vi "acquire_2_b.vi"() -> ()   [LabVIEW 2023]
panel:
  in  "stop":bool
  out "Waveform Chart":i32(graph)
  out "error out":errorcluster
  in  "error in (no error)":errorcluster
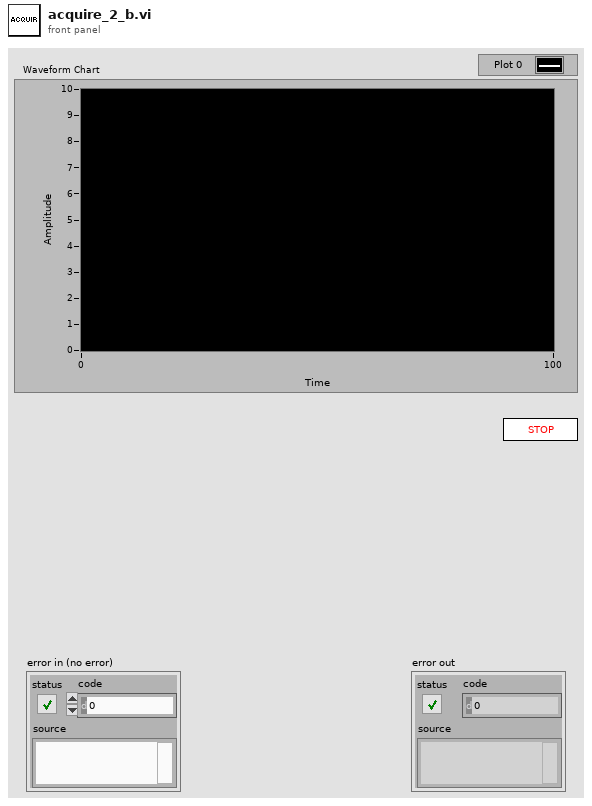
[diagram p1: front panel]
types:
  T1 = enum32{"Bad", "Idle", "Run top level", "Running"}
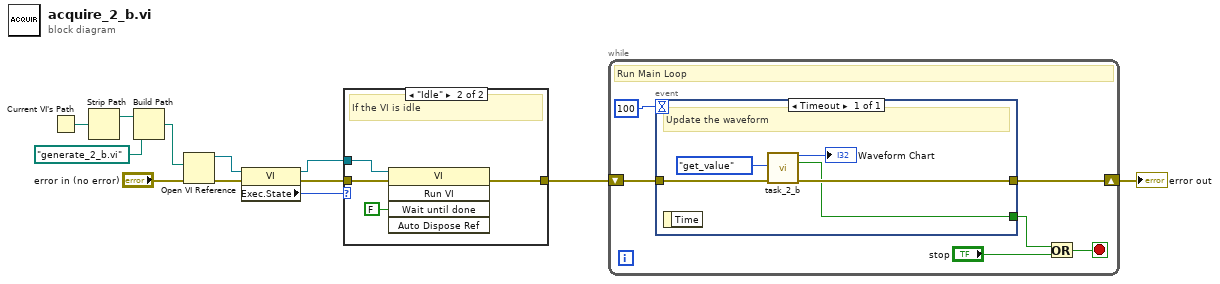
[diagram p0: block diagram]
diagram:
  n1 = Current VI's Path() -> (path=w8:path)
  n2 = Strip Path(path=w8) -> (stripped path=w9:path)  [unwired: 1 out]
  n3 = Build Path(base path=w9, name or relative path=path "generate_2_b.vi") -> (appended path=w10:path)
  n4 = Open VI Reference(vi path=w10, error in (no error)="error in (no error)") -> (vi reference=w11:refnum<vi>, error out=w12:errorcluster)  [unwired: 4 in]
  n5 = property class="VI"(reference=w11, error in=w12) -> (reference out=w1:refnum<vi>, error out=w3:errorcluster, "Exec.State"=w4:T1)
  n6 = case shown="\"Idle\"" w4 {
    tunnel: w3 -> [w13 w17]
    tunnel: [w13 w16] -> w2
    tunnel: w1 -> [_ w15]
    frame "Running", Default {
      # "If the VI is running"
    }
    frame "Idle" {
      # "If the VI is idle"
      n7 = invoke class="VI" method="Run VI"(reference=w15, error in=w17, "Wait until done"=FALSE ("Wait Until Done")) -> (error out=w16:errorcluster)  [unwired: 2 in, 4 out]
    }
  }
  n8 = while {
    shift-right: [w21] -> w5
    shift-left: w2 -> [w22]
    stop <- w20 stop-if-true
    # "Run Main Loop"
    n9 = event shown="[0] Timeout" {
      selector: _ -> [_]
      dyn-events: _ -> [_]
      timeout: 100 -> [_]
      tunnel: w22 -> [w28]
      tunnel: [w27] -> w21
      tunnel: [w24] -> w18
      event Timeout {
        # "Update the waveform"
        n10 = event-data() -> ()  [unwired: 1 in, 1 out]
        n11 = call "task_2_b.vi"("Operation"=enum16{"get_value", "set_value", "Initialize"}."get_value", "error constant"=w28) -> ("data 2"=→"Waveform Chart":i32, "Stop 2"=w24:bool, "error IO"=w27:errorcluster)  [unwired: 11 in]
      }
    }
    n12 = Or(x=w18, y="stop") -> (x .or. y?=w20:bool)
  }
  "error out" <- w5
